vi "VNA Stream.vi"(8 "error in":errorcluster, 10 "S-Parameter Graph":refnum<vi>, 11 "Acquire?":refnum<vi>) -> (0 "error out":errorcluster)   [LabVIEW 2023]
uses:
  controls/SData.ctl
  LibreVNA/Types/Trace Enum.ctl
  LibreVNA/LibreVNA.lvclass
panel:
  out "Time":timestamp
  out "Log":bool
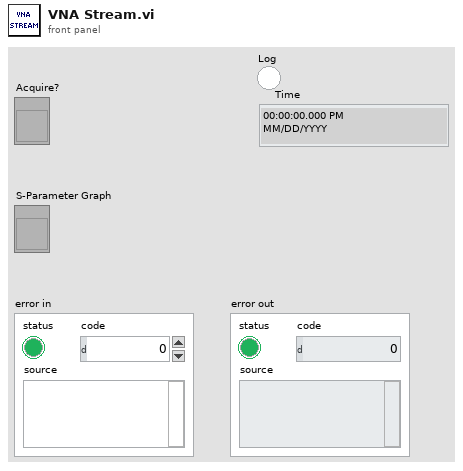
[diagram p1: front panel]
types:
  T1 = typedef "LibreVNA.lvclass/Trace Enum.ctl" = enum16{"S11", "S12", "S21", "S22"}
  T2 = typedef "SData.ctl" = cluster{"Time Stamp":timestamp, "Array":dbl[][], "Temp(C)":dbl}
  T3 = typedef "UI Data.ctl" = cluster{"session":refnum<class "Modbus Master.lvclass">, "IsOpen":bool, "Timeout (ms)":i32, "TempFile":path, "LogStartTime":timestamp, "LibreVNA":refnum<class "LibreVNA.lvclass">, "VNAOpen":bool, "TempSP":dbl, "ActualTemp":dbl, "FileSaved":bool, "PIDOutput":dbl, "VNALogOpt":refnum<vi>, "PartName":string, "ComPort":refnum<visa-resource-name>, "S-Param Data":dbl[][], "VNADataFile - TDMS":path}
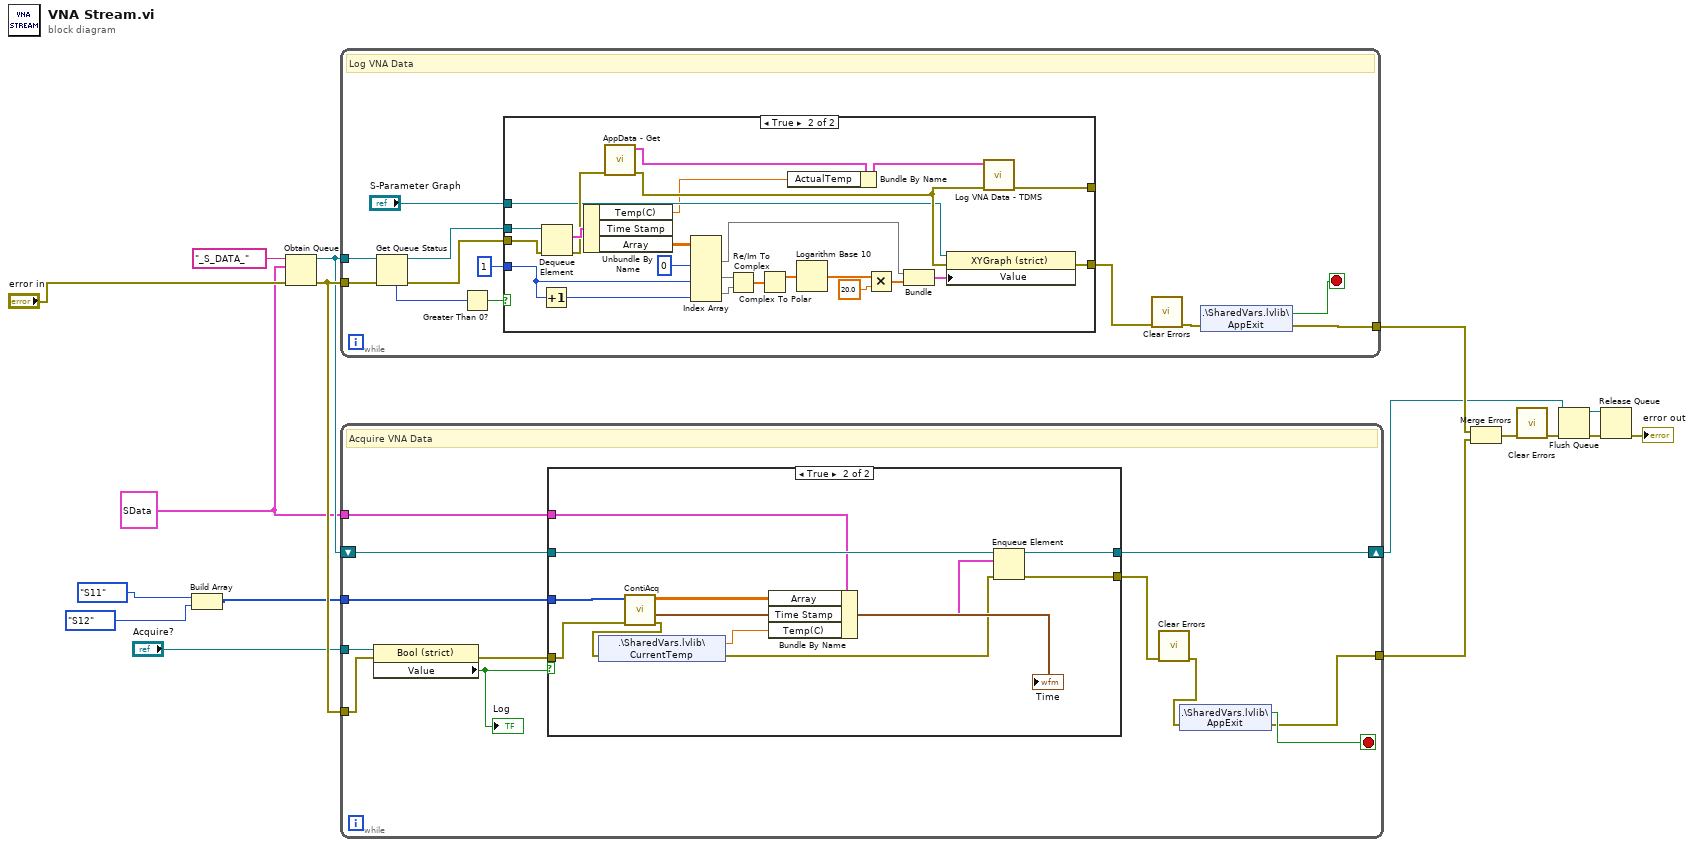
[diagram p0: block diagram]
diagram:
  w1 = T2 {"Time Stamp"=timestamp(0 s since 1904-01-01), "Array"=[], "Temp(C)"=0.0} ("S-Data")
  n1 = Build Array(Trace_Enum."S11" ("Trace Name"), Trace_Enum."S12" ("Trace Name")) -> (w2:T1[])
  n2 = Obtain Queue(name (unnamed)="_S_DATA_", element data type=w1, error in (no error)="error in") -> (queue out=w16:refnum<queue>, error out=w17:errorcluster)  [unwired: 2 in, 1 out]
  n3 = while {
    tunnel: w16 -> [w28]
    tunnel: w17 -> [w27]
    tunnel: [w21] -> w14
    stop <- w22 stop-if-true
    # "Log VNA Data"
    n4 = Get Queue Status(queue=w28, error in (no error)=w27) -> (queue out=w26:refnum<queue>, error out=w25:errorcluster, # elements in queue=w29:i32)  [unwired: 1 in, 5 out]
    n5 = Greater Than 0?(x=w29) -> (x > 0?=w24:bool)
    n6 = case shown="True" w24 {
      tunnel: w26 -> [_ w44]
      tunnel: w25 -> [w30 w43]
      tunnel: 1 ("index (col)") -> [_ w42]
      tunnel: [w30 w38] -> w20
      tunnel: [_ w36] -> _
      tunnel: "S-Parameter Graph" -> [_ w33]
      frame False {
      }
      frame True {
        n7 = Increment(x=w42) -> (x+1=w45:i32)
        n8 = Dequeue Element(queue=w44, error in (no error)=w43) -> (element=w50:T2, error out=w35:errorcluster)  [unwired: 1 in, 2 out]
        n9 = Unbundle By Name(w50) -> ("Temp(C)"=w31:dbl, "Array"=w49:dbl[][])  [unwired: 1 out]
        n10 = call "AppData - Get.vi"("error in"=w35) -> ("error out"=w34:errorcluster, "Data Out"=w37:T3)  [unwired: 5 in]
        n11 = Index Array(array=w49, index (col) #1=0 ("disabled index (col)"), index (col) #2=w42, index (col) #3=w45) -> (element #1=w41:dbl[], element #2=w48:dbl[], element #3=w47:dbl[])  [unwired: 3 in]
        n12 = Re/Im To Complex(1:w47, 2:w48) -> (0:w52:cdb[])
        n13 = Complex To Polar(r * e^(i*theta)=w52) -> (r=w53:dbl[])  [unwired: 1 out]
        n14 = Bundle By Name(cluster=w37, "ActualTemp"=w31) -> (w32:T3)
        n15 = Logarithm Base 10(1:w53) -> (0:w54:dbl[])
        n16 = Multiply(x=w54, y=20.0) -> (x*y=w40:dbl[])
        n17 = Bundle("Array"=w41, w40) -> (w39:cluster{"Array":dbl[], dbl[]})  [unwired: 1 in]
        n18 = property on="Property Node" class="XYGraph (strict)"(reference=w33, error in=w34, "Value"=w39) -> (error out=w38:errorcluster)  [unwired: 1 out]
        n19 = call "Log VNA Data - TDMS.vi"("error in (no error)"=w34, "Data in"=w32) -> ("error out"=w36:errorcluster)  [unwired: 4 in, 1 out]
      }
    }
    n20 = call <vilib>:"Clear Errors.vi"("error in (no error)"=w20) -> ("error out"=w19:errorcluster)  [unwired: 5 in, 1 out]
    n21 = shared-variable ".\\SharedVars.lvlib\\AppExit"(error in=w19) -> (w22:bool, error out=w21:errorcluster)
  }
  n22 = while {
    tunnel: w17 -> [w61]
    shift-right: [w64] -> w10
    shift-left: w16 -> [w65]
    tunnel: [w63] -> w13
    tunnel: "Acquire?" -> [w62]
    tunnel: w2 -> [w58]
    tunnel: w1 -> [w57]
    stop <- w66 stop-if-true
    # "Acquire VNA Data"
    n23 = property class="Bool (strict)"(reference=w62, error in=w61) -> (error out=w59:errorcluster, "Value"=w60:bool)  [unwired: 1 out]
    "Log" <- w60
    n24 = case shown="True" w60 {
      tunnel: w65 -> [w68 w80]
      tunnel: [w68 w72] -> w64
      tunnel: w59 -> [w67 w78]
      tunnel: w58 -> [_ w79]
      tunnel: w57 -> [_ w77]
      tunnel: [w67 w69] -> w56
      frame False {
      }
      frame True {
        n25 = call "ContiAcq.vi"("error in (no error)"=w78, "Array"=w79) -> ("error out"=w73:errorcluster, "Time"=w75:timestamp, "SData"=w76:dbl[][])  [unwired: 3 in]
        "Time" <- w75
        n26 = shared-variable ".\\SharedVars.lvlib\\CurrentTemp"(error in=w73) -> (w74:dbl, error out=w70:errorcluster)
        n27 = Bundle By Name(cluster=w77, "Array"=w76, "Time Stamp"=w75, "Temp(C)"=w74) -> (w71:T2)
        n28 = Enqueue Element(queue=w80, element=w71, error in (no error)=w70) -> (queue out=w72:refnum<queue>, error out=w69:errorcluster)  [unwired: 1 in, 1 out]
      }
    }
    n29 = call <vilib>:"Clear Errors.vi"("error in (no error)"=w56) -> ("error out"=w55:errorcluster)  [unwired: 5 in, 1 out]
    n30 = shared-variable ".\\SharedVars.lvlib\\AppExit"(error in=w55) -> (w66:bool, error out=w63:errorcluster)
  }
  n31 = Merge Errors(w14, w13) -> (w12:errorcluster)
  n32 = call <vilib>:"Clear Errors.vi"("error in (no error)"=w12) -> ("error out"=w11:errorcluster)  [unwired: 5 in, 1 out]
  n33 = Flush Queue(queue=w10, error in (no error)=w11) -> (queue out=w9:refnum<queue>, error out=w8:errorcluster)  [unwired: 1 out]
  n34 = Release Queue(queue=w9, error in (no error)=w8) -> (error out=→"error out":errorcluster)  [unwired: 1 in, 2 out]
